vi "from string.vi"(8 "error in":errorcluster, 9 "channel data":string, 10 "identifier":string, 11 "channel in":refnum<class "TBM channel.lvclass">) -> (0 "error out":errorcluster, 3 "channel out":refnum<class "TBM channel.lvclass">)   [LabVIEW 2013, in "TBM channel.lvclass"]
uses:
  TBM channel.lvclass
  <vilib>/NI/Tag Bus/tag/Data Type.ctl
  channel classification.ctl
  TBM channel.lvclass/TBM channel.ctl
  <vilib>/NI/Tag Bus/tag/tag descriptor.lvclass/tag descriptor.ctl
  <vilib>/NI/Tag Bus/tag/tag descriptor.lvclass
  <vilib>/NI/Configuration Framework/serializable configuration/NISE_CEF_serializable configuration.lvclass
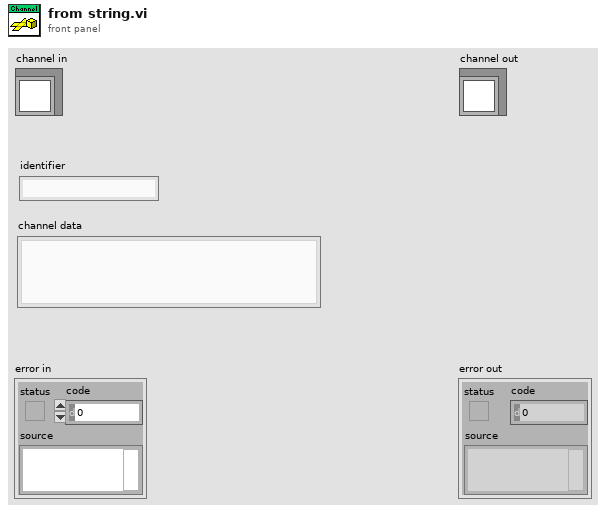
[diagram p1: front panel]
types:
  T1 = typedef "TBM channel.lvclass/channel classification.ctl" = enum16{"input data", "output data", "processing parameter", "processing result"}
  T2 = typedef "tag bus.lvlib/tag descriptor.lvclass/Data Type.ctl" = enum16{"Double", "Single", "I64", "I32", "I16", "I8", "U64", "U32", "U16", "U8", "Boolean", "String", "Array of Double", "Array of Single", "Array of I64", "Array of I32", "Array of I16", "Array of I8", "Array of U64", "Array of U32", "Array of U16", "Array of U8", "Array of Boolean", "Array of String"}
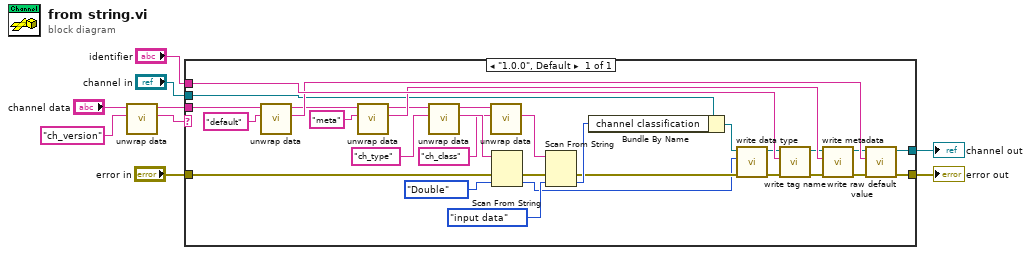
[diagram p0: block diagram]
diagram:
  n1 = call <vilib>:"unwrap data.vi"("identifier"="ch_version", "data to unwrap"="channel data") -> ("unwrapped data"=w1:string, "remaining string"=w3:string)  [unwired: 8 in]
  n2 = case shown="\"1.0.0\", Default" w1 {
    tunnel: [w39] -> w9
    tunnel: "identifier" -> [w38]
    tunnel: "channel in" -> [w19]
    tunnel: [w17] -> w6
    tunnel: w3 -> [w13]
    tunnel: "error in" -> [w12]
    frame "1.0.0", Default {
      n3 = call <vilib>:"unwrap data.vi"("identifier"="default", "data to unwrap"=w13) -> ("unwrapped data"=w32:string, "remaining string"=w22:string)  [unwired: 8 in]
      n4 = call <vilib>:"unwrap data.vi"("identifier"="meta", "data to unwrap"=w22) -> ("unwrapped data"=w31:string, "remaining string"=w26:string)  [unwired: 8 in]
      n5 = call <vilib>:"unwrap data.vi"("identifier"="ch_type", "data to unwrap"=w26) -> ("unwrapped data"=w33:string, "remaining string"=w25:string)  [unwired: 8 in]
      n6 = call <vilib>:"unwrap data.vi"("identifier"="ch_class", "data to unwrap"=w25) -> ("unwrapped data"=w35:string)  [unwired: 8 in, 1 out]
      n7 = Scan From String(input string=w33, error in=w12, default 1=Data_Type."Double" ("data type")) -> (error out=w10:errorcluster, output 1=w11:T2)  [unwired: 2 in, 2 out]
      n8 = Scan From String(input string=w35, error in=w10, default 1=channel_classification."input data" ("channel classification")) -> (error out=w18:errorcluster, output 1=w37:T1)  [unwired: 2 in, 2 out]
      n9 = Bundle By Name(cluster=w19, "channel classification"=w37) -> (w20:refnum<class "TBM channel.lvclass">)
      n10 = call <vilib>:"write data type.vi"("error in"=w18, "data type"=w11, "system tag in"=w20) -> ("error out"=w14:errorcluster, "system tag out"=w21:refnum<class "TBM channel.lvclass">)  [unwired: 7 in]
      n11 = call <vilib>:"write tag name.vi"("error in"=w14, "name"=w38, "system tag in"=w21) -> ("error out"=w15:errorcluster, "system tag out"=w29:refnum<class "TBM channel.lvclass">)  [unwired: 7 in]
      n12 = call <vilib>:"write metadata.vi"("error in"=w15, "metadata"=w31, "system tag in"=w29) -> ("error out"=w16:errorcluster, "system tag out"=w30:refnum<class "TBM channel.lvclass">)  [unwired: 7 in]
      n13 = call <vilib>:"write raw default value.vi"("error in"=w16, "raw default"=w32, "system tag in"=w30) -> ("error out"=w17:errorcluster, "system tag out"=w39:refnum<class "TBM channel.lvclass">)  [unwired: 7 in]
    }
  }
  "error out" <- w6
  "channel out" <- w9
